vi "Read High Limit.vi"(8 "error in":errorcluster, 11 "Has Control Limits in":refnum<class "Has Control Limits.lvclass">) -> (0 "error out":errorcluster, 2 "high limit":dbl, 3 "Has Control Limits out":refnum<class "Has Control Limits.lvclass">)   [LabVIEW 2020, in "PV Access.lvlib" / "PV Data.lvlib" / "Has Control Limits.lvclass"]
uses:
  Has Control Limits.lvclass
  182da66a-f6ee-47d3-9b05-9cecdf4c7a27.vi
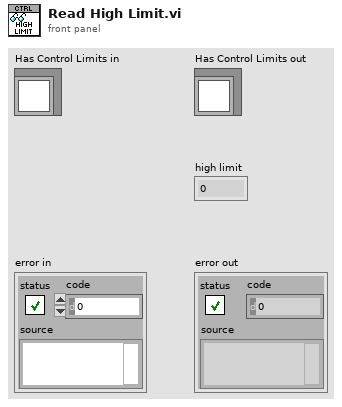
[diagram p1: front panel]
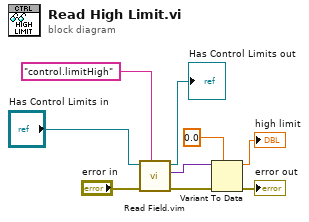
[diagram p0: block diagram]
diagram:
  n1 = call "Read Field.vim"("field"="control.limitHigh" ("element name"), "error in"="error in", "Base Interface in"="Has Control Limits in") -> ("error out"=w4:errorcluster, "value"=w3:variant, "Base Interface out"=→"Has Control Limits out":refnum<class "Has Control Limits.lvclass">)  [unwired: 6 in]
  n2 = Variant To Data(error in=w4, type=0.0, Variant=w3) -> (data=→"high limit":dbl, error out=→"error out":errorcluster)
